vi "Test TDMS dynamic data.vi"() -> ()   [LabVIEW 2016]
uses:
  <vilib>/express/express signal manip/GetorSetDDTAttributes/Shared VIs/TimeType.ctl
  <vilib>/express/express signal manip/GetorSetDDTAttributes/Shared VIs/XDimension.ctl
  <vilib>/express/express signal manip/GetorSetDDTAttributes/Shared VIs/XDimension Enum to String.vi
  <vilib>/express/express signal manip/GetorSetDDTAttributes/Shared VIs/TimeMode Enum to Boolean.vi
  <vilib>/express/express shared/transition.llb/Dynamic To Waveform Array.vi
  <vilib>/express/express signal manip/GetorSetDDTAttributes/Set DDT Attributes/SetT0.vi
  <vilib>/express/express signal manip/GetorSetDDTAttributes/Set DDT Attributes/sub Set StartTimeStamp.vi
  <vilib>/express/express shared/transition.llb/Waveform Array To Dynamic.vi
  <vilib>/Waveform/WDTOps.llb/WDT Get Waveform Time Array DBL.vi
  <vilib>/express/express signal manip/GetorSetDDTAttributes/Set DDT Attributes/Set DDT Properties.xnode
  <vilib>/express/express signal manip/GetorSetDDTAttributes/Shared VIs/GetSetShared.lvlib
  <vilib>/express/express signal manip/GetorSetDDTAttributes/Set DDT Attributes/Set DDT Attributes.lvlib
panel:
  out "Waveform Graph 2":waveform(dbl)(graph)
  in  "WFRM  Timestamp 2":timestamp
  in  "Start Timestamp 2":timestamp
  in  "Timestamp 2":timestamp
  out "names":string[](array[string])
  out "values":variant[](array[variant])
  in  "dt":dbl
  in  "WFRM  Timestamp":timestamp
  out "Waveform Graph":waveform(dbl)(graph)
  in  "X Dimension":T1
  in  "Unit":string
  in  "Start Timestamp":timestamp
  in  "Timestamp":timestamp
  in  "Time Mode":T2
  in  "Signal Name":string
  in  "File Path Control":path=path "C:/Data/test.tdms"
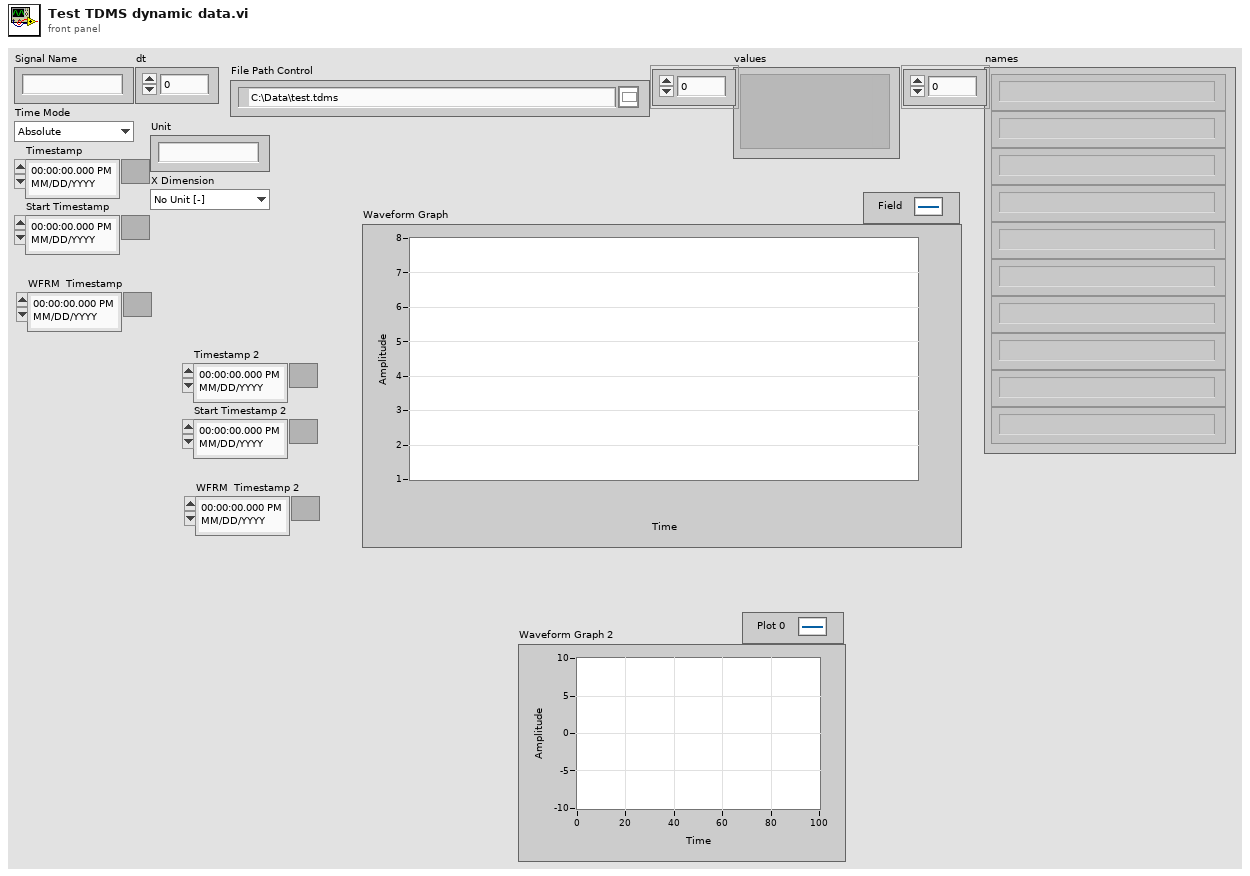
[diagram p1: front panel]
types:
  T1 = typedef "GetSetShared.lvlib/XDimension.ctl" = enum16{"No Unit [-]", "Time [sec]", "Frequency [Hz]"}
  T2 = typedef "GetSetShared.lvlib/TimeType.ctl" = enum16{"Absolute", "Relative"}
  T3 = enum16{"open", "open or create", "create or replace", "create", "open (read-only)"}
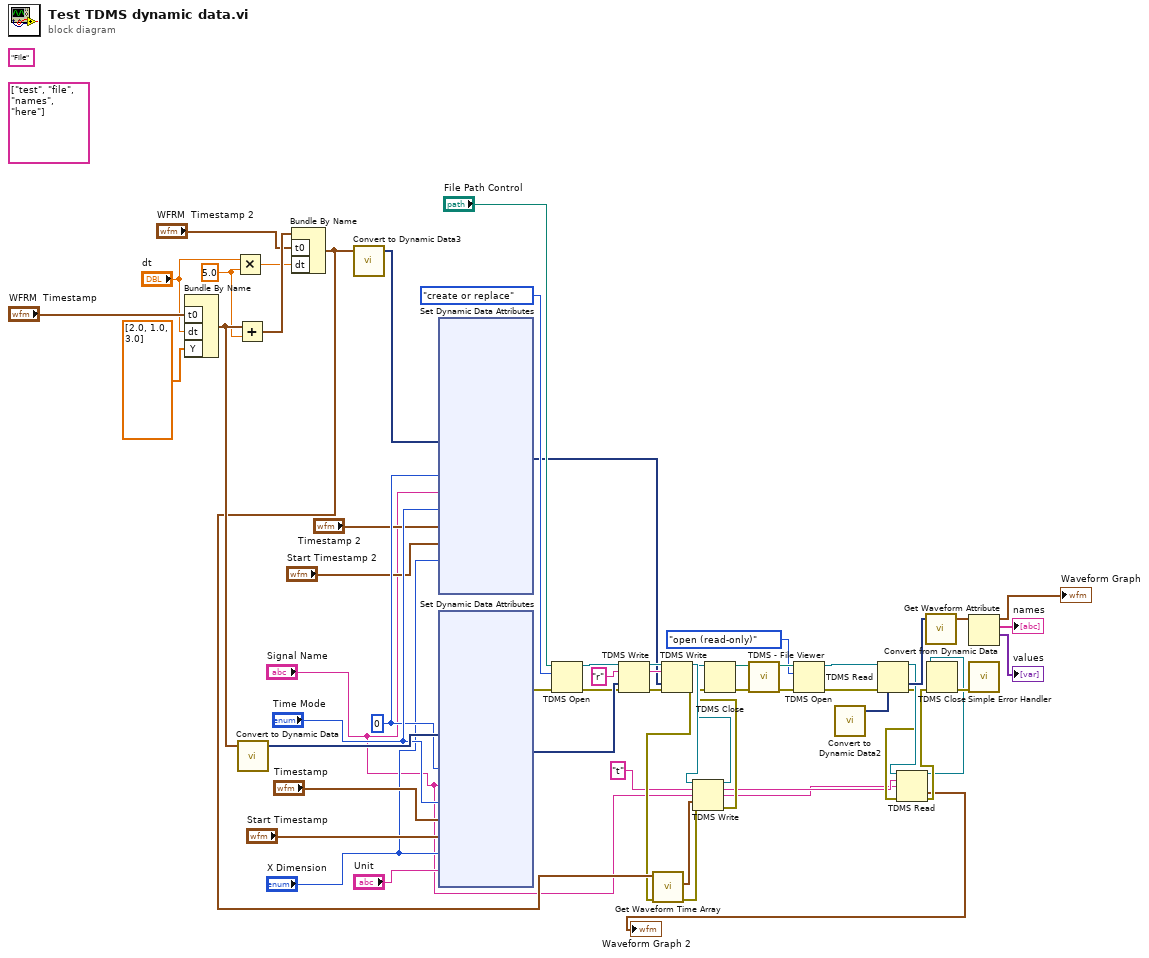
[diagram p0: block diagram]
diagram:
  w20 = 5.0 ("y")
  w24 = 0 ("Signal Index")
  (unwired) string[] ["test", "file", "names", "here"]
  (unwired) "File"
  n1 = Bundle By Name("t0"="WFRM  Timestamp", "dt"="dt", "Y"=dbl[] [2.0, 1.0, 3.0]) -> (w27:waveform(dbl))  [unwired: 1 in]
  n2 = Multiply(x="dt", y=w20) -> (x*y=w21:dbl)
  n3 = Add(x=w27, y=w20) -> (x+y=w26:waveform(dbl))
  n4 = call "Convert to Dynamic Data"("Waveform"=w27) -> ("Dynamic Data Type"=w47:dynamicdata)  [unwired: 3 in]
  n5 = Bundle By Name(cluster=w26, "t0"="WFRM  Timestamp 2", "dt"=w21) -> (w13:waveform(dbl))
  n6 = call "Convert to Dynamic Data3"("Waveform"=w13) -> ("Dynamic Data Type"=w29:dynamicdata)  [unwired: 3 in]
  n7 = xnode "Set Dynamic Data Attributes"("Signals In"=w29, "Signal Index"=w24, "Signal Name"="Signal Name", "Time Mode"="Time Mode", "Timestamp"="Timestamp 2", "Start Timestamp"="Start Timestamp 2", "X Dimension"="X Dimension") -> ("Signals Out"=w25:dynamicdata)  [unwired: 2 in, 1 out]
  n8 = xnode "Set Dynamic Data Attributes"("Signals In"=w47, "Signal Index"=w24, "Signal Name"="Signal Name", "Time Mode"="Time Mode", "Timestamp"="Timestamp", "Start Timestamp"="Start Timestamp", "X Dimension"="X Dimension", "Unit"="Unit") -> ("Signals Out"=w43:dynamicdata, "error out"=w39:errorcluster)  [unwired: 1 in]
  n9 = TDMS Open(8:w39, 10:T3."create or replace" ("operation (0:open)"), 11:"File Path Control") -> (0:w40:errorcluster, 3:w58:refnum<k34>)  [unwired: 4 in]
  n10 = TDMS Write(0:w58, 5:"r" ("group name"), 9:w43, 11:w40) -> (4:w32:refnum<k34>, 6:w31:string, 15:w49:errorcluster)  [unwired: 2 in, 1 out]
  n11 = TDMS Write(0:w32, 5:w31, 9:w25, 11:w49) -> (4:w16:refnum<k34>, 15:w10:errorcluster)  [unwired: 2 in, 2 out]
  n12 = call-poly <vilib>:"Get Waveform Time Array.vi"("error in (no error)"=w10, "waveform in"=w13) -> ("error out"=w11:errorcluster, "X array"=w12:timestamp[])  [unwired: 8 in]
  n13 = TDMS Write(0:w16, 5:"t" ("group name"), 7:"Signal Name", 9:w12, 11:w11) -> (4:w15:refnum<k34>, 6:w3:string, 8:w2:string, 15:w14:errorcluster)  [unwired: 1 in]
  n14 = TDMS Close(8:w14, 11:w15) -> (0:w56:errorcluster, 3:w55:path)
  n15 = call <vilib>:"TDMS - File Viewer.vi"("error in (no error)"=w56, "file path"=w55) -> ("error out"=w54:errorcluster, "file path out"=w53:path)  [unwired: 4 in]
  n16 = TDMS Open(8:w54, 10:T3."open (read-only)" ("operation (0:open)"), 11:w53) -> (0:w51:errorcluster, 3:w42:refnum<k34>)  [unwired: 4 in]
  n17 = call "Convert to Dynamic Data2"() -> ("Dynamic Data Type"=w41:dynamicdata)  [unwired: 4 in]
  n18 = TDMS Read(0:w42, 11:w51, 12:w41) -> (4:w7:refnum<k34>, 10:w37:dynamicdata, 15:w6:errorcluster)  [unwired: 5 in, 3 out]
  n19 = TDMS Read(0:w7, 5:w3, 7:w2, 11:w6) -> (4:w4:refnum<k34>, 10:→"Waveform Graph 2":waveform(dbl), 15:w5:errorcluster)  [unwired: 4 in, 3 out]
  n20 = call "Convert from Dynamic Data"("Dynamic Data Type"=w37) -> ("Waveform"=w33:waveform(dbl))  [unwired: 3 in]
  n21 = TDMS Close(8:w5, 11:w4) -> (0:w50:errorcluster)  [unwired: 1 out]
  n22 = Get Waveform Attribute(7:w33) -> (1:→"values":variant[], 2:→"names":string[], 3:→"Waveform Graph":waveform(dbl))  [unwired: 3 in, 1 out]
  n23 = call <vilib>:"Simple Error Handler.vi"("error in (no error)"=w50) -> ()  [unwired: 4 in, 5 out]
